vi "Timeout Eating.vi"(8 "error in (no error)":errorcluster, 11 "Philosopher in":refnum<class "Philosopher.lvclass">) -> (0 "error out":errorcluster, 3 "Philosopher out":refnum<class "Philosopher.lvclass">)   [LabVIEW 2023, in "Philosopher.lvlib" / "Philosopher.lvclass"]
uses:
  Philosopher.lvclass
  C:/Program Files (x86)/National Instruments/LabVIEW 2023/vi.lib/ActorFramework/Actor/Actor.lvclass
  Philosopher Messages/Timeout Thinking/Timeout Thinking Msg.lvclass
  C:/Program Files (x86)/National Instruments/LabVIEW 2023/vi.lib/ActorFramework/Message/Message.lvclass
  <vilib>/ActorFramework/Actor/Actor.lvclass/Actor.ctl
  <vilib>/ActorFramework/Message Enqueuer/Message Enqueuer.lvclass/Message Enqueuer.ctl
  Philosopher.lvclass/Philosopher.ctl
  Table/Table Messages/Done Eating Msg/Done Msg.lvclass/Done Msg.ctl
  <vilib>/ActorFramework/Message Enqueuer/Enqueue.vi
  <vilib>/ActorFramework/Message Enqueuer/Init from Existing Queue.vi
  Table/Table Messages/Done Eating Msg/Done Msg.lvclass
  <vilib>/Utility/LVClass/Get LV Class Name.vi
  <resource>/AFDebug/Generate Trace for Message.vi
  <vilib>/ActorFramework/Message Priority Queue/Priority Enqueue.vi
  <vilib>/ActorFramework/Message Enqueuer/Message Enqueuer.lvclass
  <vilib>/ActorFramework/Actor/Actor.lvclass
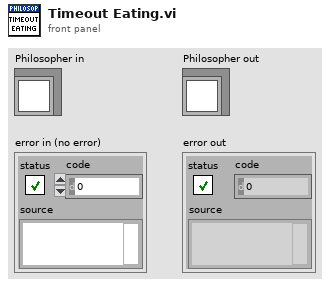
[diagram p1: front panel]
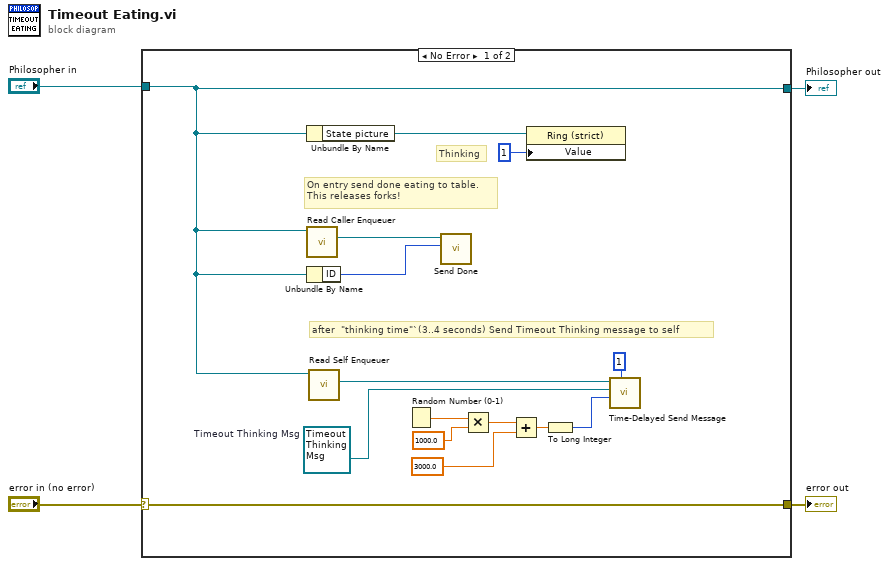
[diagram p0: block diagram]
diagram:
  n1 = case shown="No Error" "error in (no error)" {
    selector: "error in (no error)" -> [w19 w21]
    tunnel: [w19 w21] -> w3
    tunnel: [w6 w20] -> w1
    tunnel: "Philosopher in" -> [w6 w20]
    frame No Error {
      w9 = refnum<class "Timeout Thinking Msg.lvclass"> refnum  # Timeout Thinking Msg
      # "Thinking"
      # "On entry send done eating to table. \nThis releases forks!"
      # "after  \"thinking time\"`(3..4 seconds) Send Timeout Thinking message to self"
      n2 = Unbundle By Name(w6) -> ("State picture"=w18:refnum<vi>)
      n3 = call <vilib>:"Read Caller Enqueuer.vi"("Actor"=w6) -> ("Caller Enqueuer"=w8:refnum<class "Message Enqueuer.lvclass">)  [unwired: 10 in]
      n4 = Unbundle By Name(w6) -> ("ID"=w7:i32)
      n5 = call <vilib>:"Read Self Enqueuer.vi"("Actor"=w6) -> ("Self Enqueuer"=w10:refnum<class "Message Enqueuer.lvclass">)  [unwired: 10 in]
      n6 = Random Number (0-1)() -> (number: 0 to 1=w12:dbl)
      n7 = call "Send Done.vi"("Philosopher ID"=w7, "Message Enqueuer"=w8) -> ()  [unwired: 8 in, 2 out]
      n8 = Multiply(x=w12, y=1000.0) -> (x*y=w14:dbl)
      n9 = Add(x=w14, y=3000.0) -> (x+y=w16:dbl)
      n10 = property class="Ring (strict)"(reference=w18, "Value"=1) -> ()  [unwired: 1 in, 2 out]
      n11 = To Long Integer(number=w16) -> (32bit integer=w17:i32)
      n12 = call <vilib>:"Time-Delayed Send Message.vi"("# Copies (0 = infinite repeat)"=u32 1, "Milliseconds To Wait"=w17, "Message"=w9, "Message Enqueuer"=w10) -> ()  [unwired: 6 in, 2 out]
    }
    frame Error {
    }
  }
  "error out" <- w3
  "Philosopher out" <- w1
